vi "Write Timing Override.vi"(8 "error in (no error)":errorcluster, 10 "Period (s)":dbl, 11 "CIFTemplateNode in":refnum<class "CIFCorePlugin.lvclass">) -> (0 "error out":errorcluster, 3 "CIFTemplateNode out":refnum<class "CIFCorePlugin.lvclass">)   [LabVIEW 2021, in "CIFCorePlugin.lvclass"]
uses:
  CIFCorePlugin.lvclass
  CIFCoreCommon/Typedef/Timing Overrides.ctl
  CIFCorePlugin.lvclass/CIFCorePlugin.ctl
  CIFCoreCommon/CIFCoreCommon.lvlib
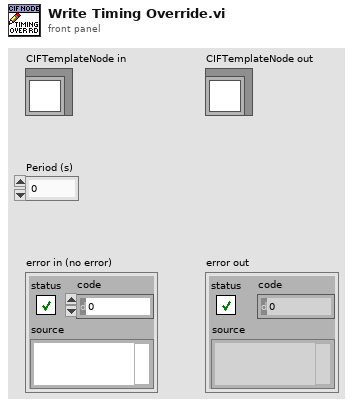
[diagram p1: front panel]
types:
  T1 = typedef "CIFCoreCommon.lvlib/Timing Overrides.ctl" = cluster{"Override Timing":bool, "Period (s)":dbl}
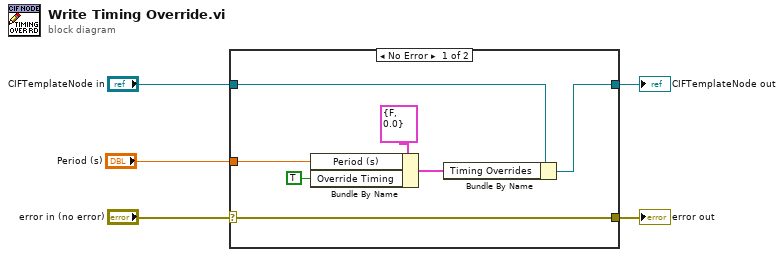
[diagram p0: block diagram]
diagram:
  n1 = case shown="No Error" "error in (no error)" {
    selector: "error in (no error)" -> [w12 w13]
    tunnel: [w12 w13] -> w4
    tunnel: [w10 w14] -> w2
    tunnel: "CIFTemplateNode in" -> [w11 w14]
    tunnel: "Period (s)" -> [w7 _]
    frame No Error {
      n2 = Bundle By Name(cluster=T1 {"Override Timing"=FALSE, "Period (s)"=0.0} ("Plugin Overrides.Timing Overrides"), "Period (s)"=w7, "Override Timing"=TRUE) -> (w9:T1)
      n3 = Bundle By Name(cluster=w11, "Timing Overrides"=w9) -> (w10:refnum<class "CIFCorePlugin.lvclass">)
    }
    frame Error {
    }
  }
  "error out" <- w4
  "CIFTemplateNode out" <- w2
